vi "PulseGeneratorFunction.vi"(1 "Channels Setup":T2(array[cluster]), 2 "Mode":T1(ring)) -> ()   [LabVIEW 2022 SP3]
uses:
  T7Examples/MODBUS/T7MOD_Write_UINT32_Register.vi
  T7Examples/MODBUS/T7MOD_Write_UINT16_Register.vi
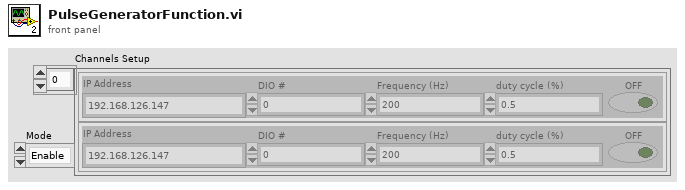
[diagram p1: front panel]
types:
  T1 = enum16{"Enable", "Disable", "Configure", "Configure and Run"}
  T2 = cluster{"IP Address":string, "DIO #":u16, "Frequency (Hz)":dbl, "duty cycle (%)":dbl, "Enable":bool}[]
  T3 = cluster{"Clock Enable":u16, "Divisor":u16, "Roll Value":u16}
  T4 = cluster{"Pulse Enable":u16, "Index":u16, "Duty Cycle":u16}
  T5 = cluster{"IP Address":string, "DIO #":u16, "Frequency (Hz)":dbl, "duty cycle (%)":dbl, "Enable":bool}
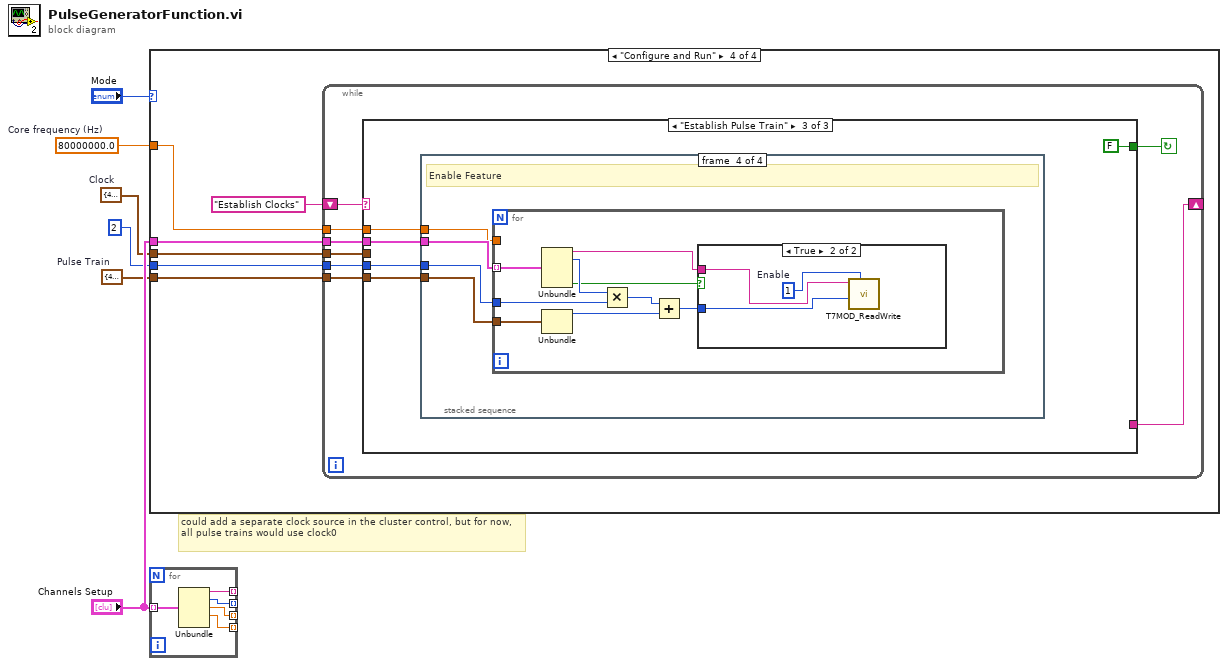
[diagram p0: block diagram]
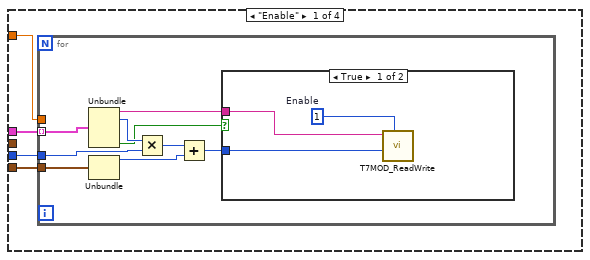
[diagram p2: hidden frame]
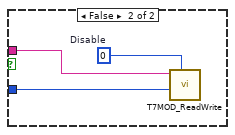
[diagram p3: hidden frame]
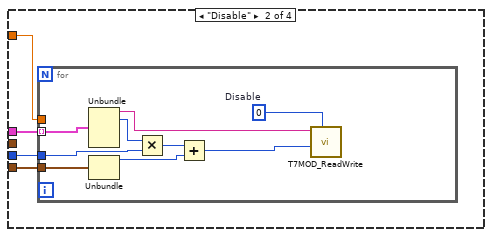
[diagram p4: hidden frame]
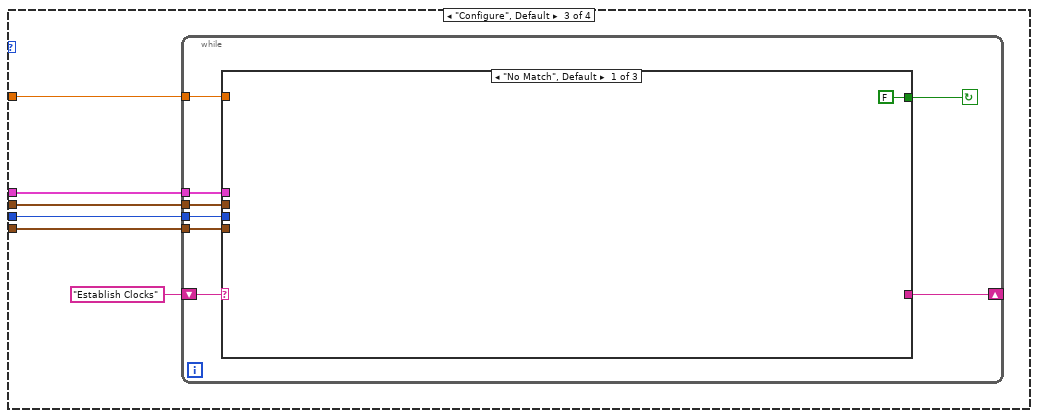
[diagram p5: hidden frame]
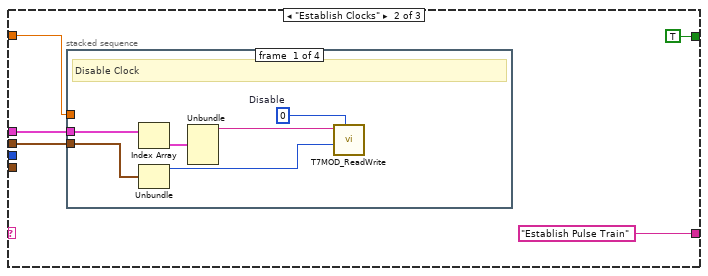
[diagram p6: hidden frame]
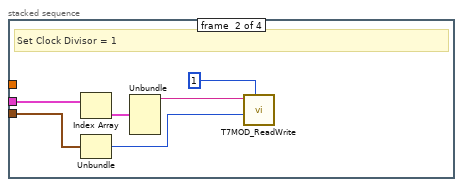
[diagram p7: hidden frame]
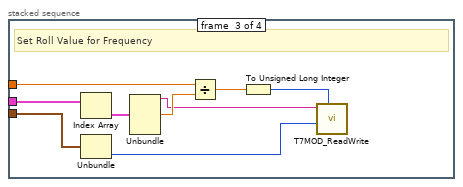
[diagram p8: hidden frame]
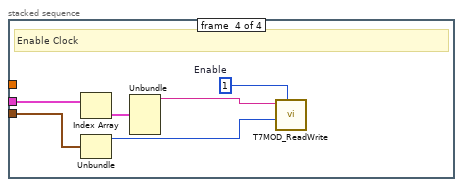
[diagram p9: hidden frame]
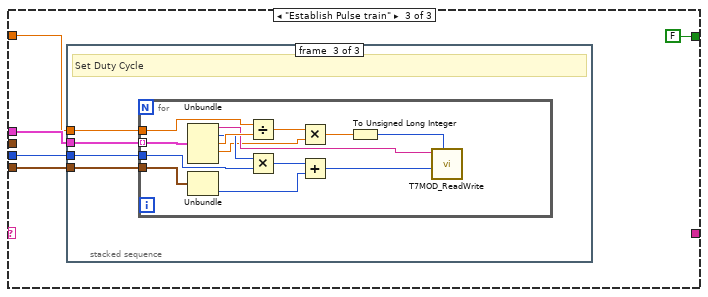
[diagram p10: hidden frame]
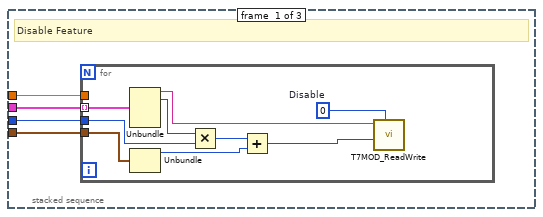
[diagram p11: hidden frame]
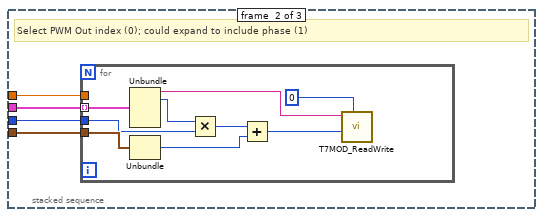
[diagram p12: hidden frame]
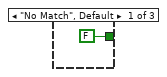
[diagram p13: hidden frame]
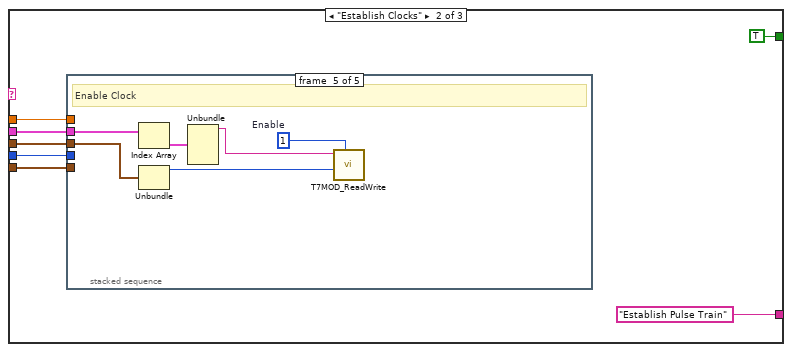
[diagram p14: hidden frame]
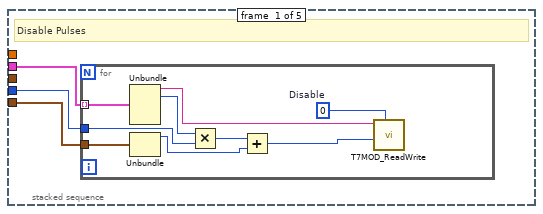
[diagram p15: hidden frame]
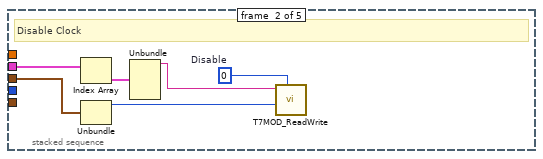
[diagram p16: hidden frame]
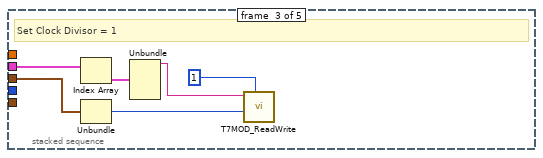
[diagram p17: hidden frame]
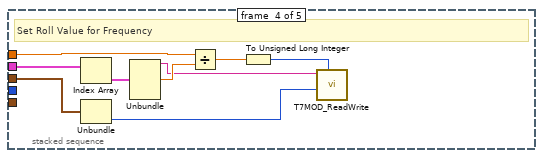
[diagram p18: hidden frame]
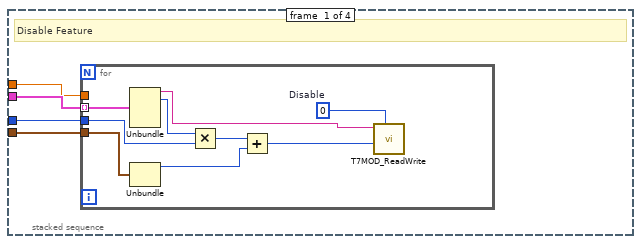
[diagram p19: hidden frame]
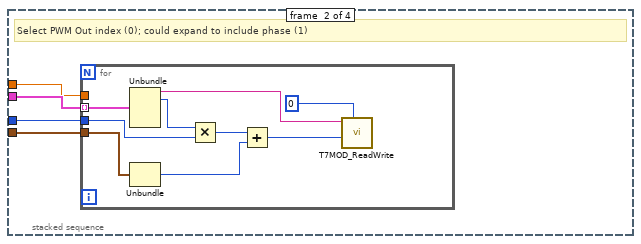
[diagram p20: hidden frame]
diagram:
  w1 = T3 {"Clock Enable"=44900, "Divisor"=44901, "Roll Value"=44904}  # Clock
  w2 = T4 {"Pulse Enable"=44000, "Index"=44100, "Duty Cycle"=44300}  # Pulse Train
  w4 = 80000000.0  # Core frequency (Hz)
  # "could add a separate clock source in the cluster control, but for now, all pulse trains would use clock0"
  n1 = case shown="\"Configure and Run\"" "Mode" {
    tunnel: "Channels Setup" -> [w10 w29 w44 w140]
    tunnel: w4 -> [w9 w28 w42 w138]
    tunnel: 2 -> [w8 w27 w41 w137]
    tunnel: w2 -> [w7 w26 w40 w136]
    tunnel: w1 -> [_ _ w39 w135]
    frame "Enable" {
      n2 = for {
        tunnel: w10 -> [w19] mode=indexing
        tunnel: w9 -> [_]
        tunnel: w7 -> [w18]
        tunnel: w8 -> [w16]
        n3 = Unbundle(w19) -> ("IP Address"=w12:string, "DIO #"=w17:u16, "Enable"=w11:bool)  [unwired: 2 out]
        n4 = Unbundle(w18) -> ("Pulse Enable"=w14:u16)  [unwired: 2 out]
        n5 = Multiply(x=w17, y=w16) -> (x*y=w15:i32)
        n6 = Add(x=w15, y=w14) -> (x+y=w13:i32)
        n7 = case shown="True" w11 {
          tunnel: w13 -> [w22 w25]
          tunnel: w12 -> [w21 w24]
          frame True {
            w20 = u32 1  # Enable
            n8 = call-poly "T7MOD_ReadWrite.vi"("UINT32 to Write"=w20, "LabJack UINT32 Register"=w22, "Remote IP Address"=w21) -> ()  [unwired: 7 in, 2 out]
          }
          frame False {
            w23 = u32 0  # Disable
            n9 = call-poly "T7MOD_ReadWrite.vi"("UINT32 to Write"=w23, "LabJack UINT32 Register"=w25, "Remote IP Address"=w24) -> ()  [unwired: 7 in, 2 out]
          }
        }
      }
    }
    frame "Disable" {
      n10 = for {
        tunnel: w29 -> [w38] mode=indexing
        tunnel: w28 -> [_]
        tunnel: w26 -> [w37]
        tunnel: w27 -> [w35]
        w30 = u32 0  # Disable
        n11 = Unbundle(w38) -> ("IP Address"=w31:string, "DIO #"=w36:u16)  [unwired: 3 out]
        n12 = Unbundle(w37) -> ("Pulse Enable"=w33:u16)  [unwired: 2 out]
        n13 = Multiply(x=w36, y=w35) -> (x*y=w34:i32)
        n14 = Add(x=w34, y=w33) -> (x+y=w32:i32)
        n15 = call-poly "T7MOD_ReadWrite.vi"("UINT32 to Write"=w30, "LabJack UINT32 Register"=w32, "Remote IP Address"=w31) -> ()  [unwired: 7 in, 2 out]
      }
    }
    frame "Configure", Default {
      n16 = while {
        tunnel: w42 -> [w51]
        tunnel: w39 -> [w50]
        tunnel: w44 -> [w49]
        tunnel: w40 -> [w48]
        tunnel: w41 -> [w47]
        shift-right: [w46] -> _
        shift-left: "Establish Clocks" -> [w52]
        stop <- w45 continue-if-true
        n17 = case shown="\"No Match\", Default" w52 {
          tunnel: w49 -> [_ w58 w90]
          tunnel: w51 -> [_ w57 w89]
          tunnel: w50 -> [_ w56 _]
          tunnel: w48 -> [_ _ w88]
          tunnel: w47 -> [_ _ w87]
          tunnel: [_ "Establish Pulse Train" _] -> w46
          tunnel: [FALSE TRUE FALSE] -> w45
          frame "No Match", Default {
          }
          frame "Establish Clocks" {
            n18 = stacked-sequence {
              tunnel: w58 -> [w60 w66 w72 w81]
              tunnel: w57 -> [_ _ w79 _]
              tunnel: w56 -> [w64 w70 w78 w85]
              frame #0 {
                w61 = u16 0  # Disable
                # "Disable Clock"
                n19 = Index Array(array=w60) -> (element=w59:T5)  [unwired: 1 in]
                n20 = Unbundle(w64) -> ("Clock Enable"=w63:u16)  [unwired: 2 out]
                n21 = Unbundle(w59) -> ("IP Address"=w62:string)  [unwired: 4 out]
                n22 = call-poly "T7MOD_ReadWrite.vi"("UINT16 to Write"=w61, "LabJack UINT16 Register"=w63, "Remote IP Address"=w62) -> ()  [unwired: 7 in, 2 out]
              }
              frame #1 {
                # "Set Clock Divisor = 1"
                n23 = Index Array(array=w66) -> (element=w65:T5)  [unwired: 1 in]
                n24 = Unbundle(w70) -> ("Divisor"=w67:u16)  [unwired: 2 out]
                n25 = Unbundle(w65) -> ("IP Address"=w69:string)  [unwired: 4 out]
                n26 = call-poly "T7MOD_ReadWrite.vi"("UINT16 to Write"=u16 1 ("Disable"), "LabJack UINT16 Register"=w67, "Remote IP Address"=w69) -> ()  [unwired: 7 in, 2 out]
              }
              frame #2 {
                # "Set Roll Value for Frequency"
                n27 = Index Array(array=w72) -> (element=w71:T5)  [unwired: 1 in]
                n28 = Unbundle(w78) -> ("Roll Value"=w75:u16)  [unwired: 2 out]
                n29 = Unbundle(w71) -> ("IP Address"=w73:string, "Frequency (Hz)"=w77:dbl)  [unwired: 3 out]
                n30 = Divide(x=w79, y=w77) -> (x/y=w76:dbl)
                n31 = To Unsigned Long Integer(number=w76) -> (unsigned 32bit integer=w74:u32)
                n32 = call-poly "T7MOD_ReadWrite.vi"("UINT32 to Write"=w74, "LabJack UINT32 Register"=w75, "Remote IP Address"=w73) -> ()  [unwired: 7 in, 2 out]
              }
              frame #3 {
                w82 = u16 1  # Enable
                # "Enable Clock"
                n33 = Index Array(array=w81) -> (element=w80:T5)  [unwired: 1 in]
                n34 = Unbundle(w85) -> ("Clock Enable"=w84:u16)  [unwired: 2 out]
                n35 = Unbundle(w80) -> ("IP Address"=w83:string)  [unwired: 4 out]
                n36 = call-poly "T7MOD_ReadWrite.vi"("UINT16 to Write"=w82, "LabJack UINT16 Register"=w84, "Remote IP Address"=w83) -> ()  [unwired: 7 in, 2 out]
              }
            }
          }
          frame "Establish Pulse train" {
            n37 = stacked-sequence {
              tunnel: w90 -> [w94 w107 w120]
              tunnel: w89 -> [w93 w106 w119]
              tunnel: w88 -> [w92 w105 w118]
              tunnel: w87 -> [w91 w104 w117]
              frame #0 {
                # "Disable Feature"
                n38 = for {
                  tunnel: w94 -> [w103] mode=indexing
                  tunnel: w93 -> [_]
                  tunnel: w92 -> [w102]
                  tunnel: w91 -> [w100]
                  w95 = u32 0  # Disable
                  n39 = Unbundle(w103) -> ("IP Address"=w96:string, "DIO #"=w101:u16)  [unwired: 3 out]
                  n40 = Unbundle(w102) -> ("Pulse Enable"=w98:u16)  [unwired: 2 out]
                  n41 = Multiply(x=w101, y=w100) -> (x*y=w99:i32)
                  n42 = Add(x=w99, y=w98) -> (x+y=w97:i32)
                  n43 = call-poly "T7MOD_ReadWrite.vi"("UINT32 to Write"=w95, "LabJack UINT32 Register"=w97, "Remote IP Address"=w96) -> ()  [unwired: 7 in, 2 out]
                }
              }
              frame #1 {
                # "Select PWM Out index (0); could expand to include phase (1)"
                n44 = for {
                  tunnel: w107 -> [w116] mode=indexing
                  tunnel: w106 -> [_]
                  tunnel: w105 -> [w115]
                  tunnel: w104 -> [w113]
                  n45 = Unbundle(w116) -> ("IP Address"=w110:string, "DIO #"=w114:u16)  [unwired: 3 out]
                  n46 = Unbundle(w115) -> ("Index"=w108:u16)  [unwired: 2 out]
                  n47 = Multiply(x=w114, y=w113) -> (x*y=w112:i32)
                  n48 = Add(x=w112, y=w108) -> (x+y=w111:i32)
                  n49 = call-poly "T7MOD_ReadWrite.vi"("UINT32 to Write"=u32 0 ("Disable"), "LabJack UINT32 Register"=w111, "Remote IP Address"=w110) -> ()  [unwired: 7 in, 2 out]
                }
              }
              frame #2 {
                # "Set Duty Cycle"
                n50 = for {
                  tunnel: w120 -> [w134] mode=indexing
                  tunnel: w119 -> [w133]
                  tunnel: w118 -> [w131]
                  tunnel: w117 -> [w129]
                  n51 = Unbundle(w134) -> ("IP Address"=w124:string, "DIO #"=w130:u16, "Frequency (Hz)"=w132:dbl, "duty cycle (%)"=w121:dbl)  [unwired: 1 out]
                  n52 = Unbundle(w131) -> ("Duty Cycle"=w127:u16)  [unwired: 2 out]
                  n53 = Divide(x=w133, y=w132) -> (x/y=w122:dbl)
                  n54 = Multiply(x=w130, y=w129) -> (x*y=w128:i32)
                  n55 = Multiply(x=w122, y=w121) -> (x*y=w123:dbl)
                  n56 = Add(x=w128, y=w127) -> (x+y=w125:i32)
                  n57 = To Unsigned Long Integer(number=w123) -> (unsigned 32bit integer=w126:u32)
                  n58 = call-poly "T7MOD_ReadWrite.vi"("UINT32 to Write"=w126, "LabJack UINT32 Register"=w125, "Remote IP Address"=w124) -> ()  [unwired: 7 in, 2 out]
                }
              }
            }
          }
        }
      }
    }
    frame "Configure and Run" {
      n59 = while {
        tunnel: w138 -> [w147]
        tunnel: w135 -> [w146]
        tunnel: w140 -> [w145]
        tunnel: w136 -> [w144]
        tunnel: w137 -> [w143]
        shift-right: [w142] -> _
        shift-left: "Establish Clocks" -> [w148]
        stop <- w141 continue-if-true
        n60 = case shown="\"Establish Pulse Train\"" w148 {
          tunnel: w145 -> [_ w156 w200]
          tunnel: w147 -> [_ w155 w199]
          tunnel: w146 -> [_ w154 _]
          tunnel: w144 -> [_ w151 w198]
          tunnel: w143 -> [_ w150 w197]
          tunnel: [_ "Establish Pulse Train" _] -> w142
          tunnel: [FALSE TRUE FALSE] -> w141
          frame "No Match", Default {
          }
          frame "Establish Clocks" {
            n61 = stacked-sequence {
              tunnel: w156 -> [w159 w170 w176 w182 w191]
              tunnel: w155 -> [_ _ _ w189 _]
              tunnel: w154 -> [_ w174 w180 w188 w195]
              tunnel: w151 -> [w158 _ _ _ _]
              tunnel: w150 -> [w157 _ _ _ _]
              frame #0 {
                # "Disable Pulses"
                n62 = for {
                  tunnel: w159 -> [w168] mode=indexing
                  tunnel: w158 -> [w167]
                  tunnel: w157 -> [w165]
                  w160 = u32 0  # Disable
                  n63 = Unbundle(w168) -> ("IP Address"=w161:string, "DIO #"=w166:u16)  [unwired: 3 out]
                  n64 = Unbundle(w167) -> ("Pulse Enable"=w163:u16)  [unwired: 2 out]
                  n65 = Multiply(x=w166, y=w165) -> (x*y=w164:i32)
                  n66 = Add(x=w164, y=w163) -> (x+y=w162:i32)
                  n67 = call-poly "T7MOD_ReadWrite.vi"("UINT32 to Write"=w160, "LabJack UINT32 Register"=w162, "Remote IP Address"=w161) -> ()  [unwired: 7 in, 2 out]
                }
              }
              frame #1 {
                w171 = u16 0  # Disable
                # "Disable Clock"
                n68 = Index Array(array=w170) -> (element=w169:T5)  [unwired: 1 in]
                n69 = Unbundle(w174) -> ("Clock Enable"=w173:u16)  [unwired: 2 out]
                n70 = Unbundle(w169) -> ("IP Address"=w172:string)  [unwired: 4 out]
                n71 = call-poly "T7MOD_ReadWrite.vi"("UINT16 to Write"=w171, "LabJack UINT16 Register"=w173, "Remote IP Address"=w172) -> ()  [unwired: 7 in, 2 out]
              }
              frame #2 {
                # "Set Clock Divisor = 1"
                n72 = Index Array(array=w176) -> (element=w175:T5)  [unwired: 1 in]
                n73 = Unbundle(w180) -> ("Divisor"=w177:u16)  [unwired: 2 out]
                n74 = Unbundle(w175) -> ("IP Address"=w179:string)  [unwired: 4 out]
                n75 = call-poly "T7MOD_ReadWrite.vi"("UINT16 to Write"=u16 1 ("Disable"), "LabJack UINT16 Register"=w177, "Remote IP Address"=w179) -> ()  [unwired: 7 in, 2 out]
              }
              frame #3 {
                # "Set Roll Value for Frequency"
                n76 = Index Array(array=w182) -> (element=w181:T5)  [unwired: 1 in]
                n77 = Unbundle(w188) -> ("Roll Value"=w185:u16)  [unwired: 2 out]
                n78 = Unbundle(w181) -> ("IP Address"=w183:string, "Frequency (Hz)"=w187:dbl)  [unwired: 3 out]
                n79 = Divide(x=w189, y=w187) -> (x/y=w186:dbl)
                n80 = To Unsigned Long Integer(number=w186) -> (unsigned 32bit integer=w184:u32)
                n81 = call-poly "T7MOD_ReadWrite.vi"("UINT32 to Write"=w184, "LabJack UINT32 Register"=w185, "Remote IP Address"=w183) -> ()  [unwired: 7 in, 2 out]
              }
              frame #4 {
                w192 = u16 1  # Enable
                # "Enable Clock"
                n82 = Index Array(array=w191) -> (element=w190:T5)  [unwired: 1 in]
                n83 = Unbundle(w195) -> ("Clock Enable"=w194:u16)  [unwired: 2 out]
                n84 = Unbundle(w190) -> ("IP Address"=w193:string)  [unwired: 4 out]
                n85 = call-poly "T7MOD_ReadWrite.vi"("UINT16 to Write"=w192, "LabJack UINT16 Register"=w194, "Remote IP Address"=w193) -> ()  [unwired: 7 in, 2 out]
              }
            }
          }
          frame "Establish Pulse Train" {
            n86 = stacked-sequence {
              tunnel: w200 -> [w204 w217 w230 w248]
              tunnel: w199 -> [w203 w216 w229 w247]
              tunnel: w198 -> [w202 w215 w228 w246]
              tunnel: w197 -> [w201 w214 w227 w245]
              frame #0 {
                # "Disable Feature"
                n87 = for {
                  tunnel: w204 -> [w213] mode=indexing
                  tunnel: w203 -> [_]
                  tunnel: w202 -> [w212]
                  tunnel: w201 -> [w210]
                  w205 = u32 0  # Disable
                  n88 = Unbundle(w213) -> ("IP Address"=w206:string, "DIO #"=w211:u16)  [unwired: 3 out]
                  n89 = Unbundle(w212) -> ("Pulse Enable"=w208:u16)  [unwired: 2 out]
                  n90 = Multiply(x=w211, y=w210) -> (x*y=w209:i32)
                  n91 = Add(x=w209, y=w208) -> (x+y=w207:i32)
                  n92 = call-poly "T7MOD_ReadWrite.vi"("UINT32 to Write"=w205, "LabJack UINT32 Register"=w207, "Remote IP Address"=w206) -> ()  [unwired: 7 in, 2 out]
                }
              }
              frame #1 {
                # "Select PWM Out index (0); could expand to include phase (1)"
                n93 = for {
                  tunnel: w217 -> [w226] mode=indexing
                  tunnel: w216 -> [_]
                  tunnel: w215 -> [w225]
                  tunnel: w214 -> [w223]
                  n94 = Unbundle(w226) -> ("IP Address"=w220:string, "DIO #"=w224:u16)  [unwired: 3 out]
                  n95 = Unbundle(w225) -> ("Index"=w218:u16)  [unwired: 2 out]
                  n96 = Multiply(x=w224, y=w223) -> (x*y=w222:i32)
                  n97 = Add(x=w222, y=w218) -> (x+y=w221:i32)
                  n98 = call-poly "T7MOD_ReadWrite.vi"("UINT32 to Write"=u32 0 ("Disable"), "LabJack UINT32 Register"=w221, "Remote IP Address"=w220) -> ()  [unwired: 7 in, 2 out]
                }
              }
              frame #2 {
                # "Set Duty Cycle"
                n99 = for {
                  tunnel: w230 -> [w244] mode=indexing
                  tunnel: w229 -> [w243]
                  tunnel: w228 -> [w241]
                  tunnel: w227 -> [w239]
                  n100 = Unbundle(w244) -> ("IP Address"=w234:string, "DIO #"=w240:u16, "Frequency (Hz)"=w242:dbl, "duty cycle (%)"=w231:dbl)  [unwired: 1 out]
                  n101 = Unbundle(w241) -> ("Duty Cycle"=w237:u16)  [unwired: 2 out]
                  n102 = Divide(x=w243, y=w242) -> (x/y=w232:dbl)
                  n103 = Multiply(x=w240, y=w239) -> (x*y=w238:i32)
                  n104 = Multiply(x=w232, y=w231) -> (x*y=w233:dbl)
                  n105 = Add(x=w238, y=w237) -> (x+y=w235:i32)
                  n106 = To Unsigned Long Integer(number=w233) -> (unsigned 32bit integer=w236:u32)
                  n107 = call-poly "T7MOD_ReadWrite.vi"("UINT32 to Write"=w236, "LabJack UINT32 Register"=w235, "Remote IP Address"=w234) -> ()  [unwired: 7 in, 2 out]
                }
              }
              frame #3 {
                # "Enable Feature"
                n108 = for {
                  tunnel: w248 -> [w257] mode=indexing
                  tunnel: w247 -> [_]
                  tunnel: w246 -> [w256]
                  tunnel: w245 -> [w254]
                  n109 = Unbundle(w257) -> ("IP Address"=w250:string, "DIO #"=w255:u16, "Enable"=w249:bool)  [unwired: 2 out]
                  n110 = Unbundle(w256) -> ("Pulse Enable"=w252:u16)  [unwired: 2 out]
                  n111 = Multiply(x=w255, y=w254) -> (x*y=w253:i32)
                  n112 = Add(x=w253, y=w252) -> (x+y=w251:i32)
                  n113 = case shown="True" w249 {
                    tunnel: w251 -> [_ w260]
                    tunnel: w250 -> [_ w259]
                    frame False {
                    }
                    frame True {
                      w258 = u32 1  # Enable
                      n114 = call-poly "T7MOD_ReadWrite.vi"("UINT32 to Write"=w258, "LabJack UINT32 Register"=w260, "Remote IP Address"=w259) -> ()  [unwired: 7 in, 2 out]
                    }
                  }
                }
              }
            }
          }
        }
      }
    }
  }
  n115 = for {
    tunnel: "Channels Setup" -> [w265] mode=indexing
    tunnel: [w264] -> _ mode=indexing
    tunnel: [w263] -> _ mode=indexing
    tunnel: [w262] -> _ mode=indexing
    tunnel: [w261] -> _ mode=indexing
    n116 = Unbundle(w265) -> ("IP Address"=w264:string, "DIO #"=w263:u16, "Frequency (Hz)"=w262:dbl, "duty cycle (%)"=w261:dbl)  [unwired: 1 out]
  }
